vi "Settings - NI 9219.vi"(8 "Error In":errorcluster) -> (0 "Error Out":errorcluster={"status"=TRUE, "code"=-200077, "source"="Property Node DAQmx Channel (arg 2) in DAQmx Create Channel (AI-Temperature-Thermocouple).vi:1->Settings - NI 9211.vi <append>\n<B>Property: </B>AI.Temp.Units\n<B>Requested Value: </B>\n<B>You Can Select: </B>Deg C, Deg F, Kelvins, Deg R, From Custom Scale\n\n<B>Channel Name: </B>Temperature\n\n<B>Task Name: </B>_unnamedTask<E>"}, 3 "Cancelled?":bool)   [LabVIEW 2011]
doc: "This VI will get settings for NI 9211 measurement."
uses:
  SubVIs/Controls/4ch.ctl
  SubVIs/Controls/TransparencyEffectOperations.ctl
  <vilib>/DAQmx/create/channels.llb/DAQmx Create Channel (AI-Temperature-Thermocouple).vi
  <vilib>/DAQmx/configure/timing.llb/DAQmx Timing (Sample Clock).vi
  Program Files/National Instruments/LabVIEW 2011/resource/objmgr/daqmx.rc
panel:
  in  "NR of Samples":i32=3
  in  "Sample Mode":i32(ring)=10123 items=["Finite Samples"=10178, "Continuous Samples"=10123, "Hardware Timed Single Point"=12522]
  in  "Rate":dbl=10.0
  in  "Unit":i32(ring)=10143 items=["Deg C"=10143, "Deg F"=10144, "Kelvins"=10325, "Deg R"=10145, "From Custom Scale"=10065]
  in  "Thermocouple Type":i32(ring)=10072 items=["J"=10072, "K"=10073, "N"=10077, "R"=10082, "S"=10085, "T"=10086, "B"=10047, "E"=10055]
  in  "CJC source":i32(ring)=10200 items=["Built-In"=10200, "Constant Value"=10116, "Channel"=10113]
  in  "Channel":T1
  in  "Min":dbl=10.0
  in  "Max":dbl=40.0
  in  "Header For Measurement File":string="Temperature CH0"
  in  "Cancel Button":bool
  in  "OK Button":bool
  # "NI 9219"
  # "Meas File Settings"
  # "Hardware Settings"
  # "Signal Input Range"
  # "Scaled Units"
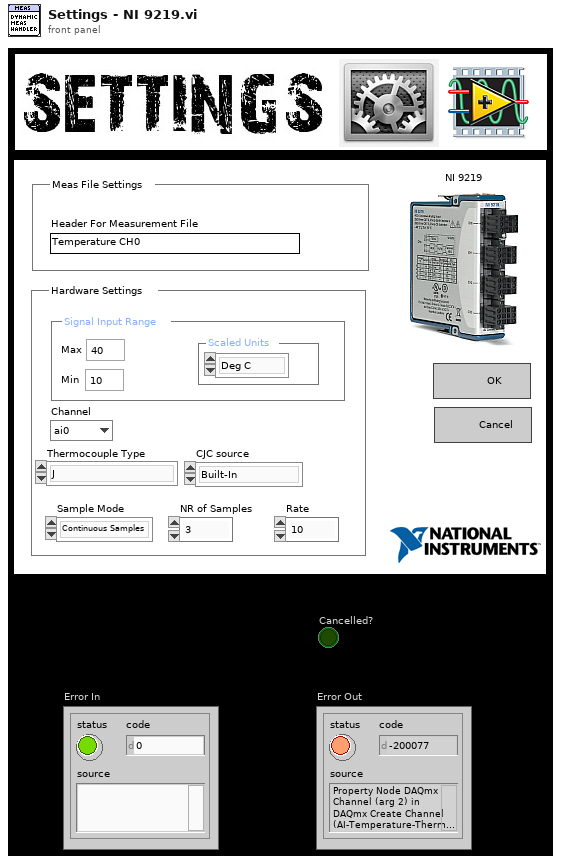
[diagram p1: front panel]
types:
  T1 = typedef "4ch.ctl" = enum16{"ai0", "ai1", "ai2", "ai3"}
  T2 = typedef "TransparencyEffectOperations.ctl" = enum16{"Show", "Hide 80%", "Hide All"}
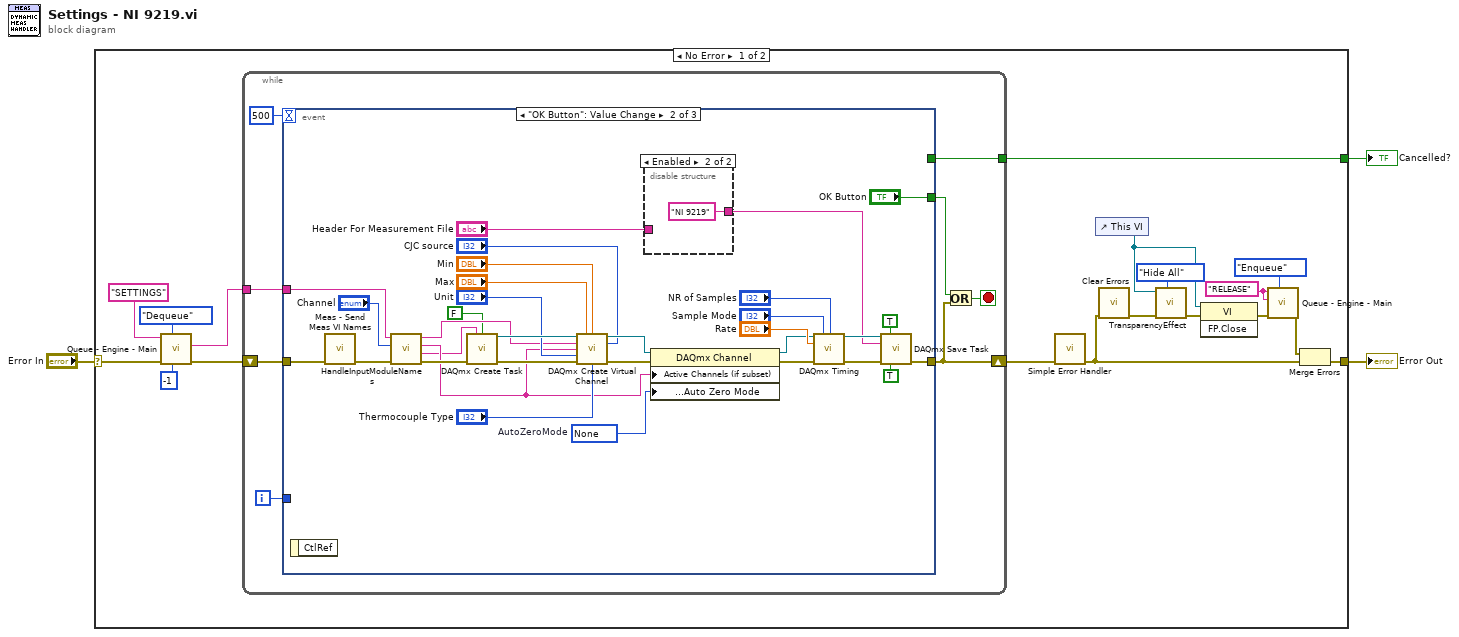
[diagram p0: block diagram]
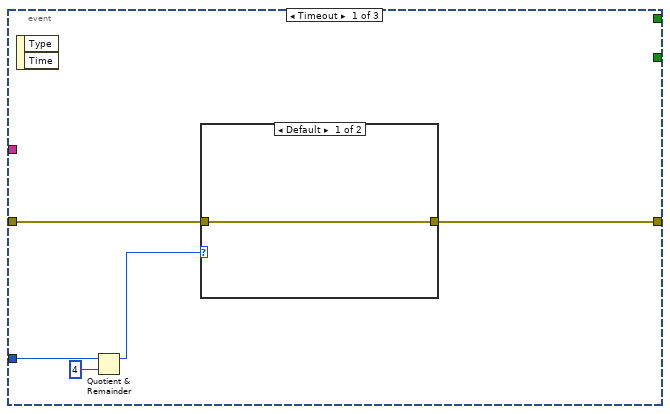
[diagram p2: hidden frame]
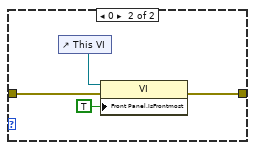
[diagram p3: hidden frame]
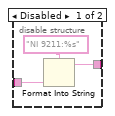
[diagram p4: hidden frame]
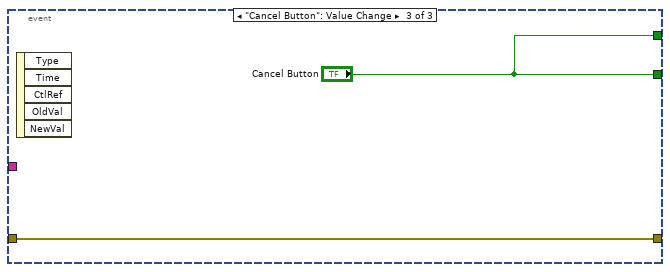
[diagram p5: hidden frame]
diagram:
  n1 = case shown="No Error" "Error In" {
    selector: "Error In" -> [w18 w78]
    tunnel: [w21 _] -> w3
    tunnel: [w4 w78] -> w2
    frame No Error {
      w10 = "RELEASE" ("Queue Data In")
      n2 = call "Queue - Engine - Main.vi"("timeout in ms (-1)"=-1, "Operation"=enum16{"Enqueue", "Dequeue", "Flush", "Release"}."Dequeue", "error in"=w18, "Queue Name In"="SETTINGS") -> ("error out"=w17:errorcluster, "Data Out"=w16:string)  [unwired: 5 in, 1 out]
      n3 = while {
        tunnel: [w29] -> w21
        shift-right: [w24] -> w5
        shift-left: w17 -> [w28]
        tunnel: w16 -> [w27]
        i -> [w25]
        stop <- w22 stop-if-true
        n4 = event shown="[1] \"OK Button\": Value Change" {
          selector: _ -> [_ _ _]
          dyn-events: _ -> [_ _ _]
          timeout: 500 -> [_ _ _]
          tunnel: [_ "OK Button" "Cancel Button"] -> w23
          tunnel: [_ _ "Cancel Button"] -> w29
          tunnel: [w33 w43 w76] -> w24
          tunnel: w28 -> [w34 w48 w76]
          tunnel: w27 -> [_ w60 _]
          tunnel: w25 -> [w32 _ _]
          event Timeout {
            n5 = event-data() -> ()  [unwired: 1 in, 2 out]
            n6 = Quotient & Remainder(x=w32, y=4) -> (x-y*floor(x/y)=w30:i32)  [unwired: 1 out]
            n7 = case shown="Default" w30 {
              tunnel: w34 -> [w35 w38]
              tunnel: [w35 w37] -> w33
              frame Default {
              }
              frame 0 {
                n8 = control-ref of="This VI"() -> (w39:refnum<vi>)
                n9 = property class="VI"(reference=w39, error in=w38, "Front Panel.IsFrontmost"=TRUE ("Front Panel Window:Is Frontmost")) -> (error out=w37:errorcluster)  [unwired: 1 out]
              }
            }
          }
          event "OK Button": Value Change {
            w69 = 10230 items=["None"=10230, "Once"=10244, "Every Sample"=10164]  # AutoZeroMode
            n10 = event-data() -> ()  [unwired: 1 in, 1 out]
            n11 = call "Meas - Send Meas VI Names.vi"("Error In"=w48) -> ("Error Out"=w47:errorcluster)  [unwired: 10 in]
            n12 = call "HandleInputModuleNames.vi"("Error In"=w47, "Channel"="Channel", "Data In"=w60) -> ("Error Out"=w62:errorcluster, "Meas Name"=w57:string, "Module and CH"=w59:string, "Channel"=w61:string)  [unwired: 5 in]
            n13 = call <vilib>:"DAQmx Create Task.vi"("new task name"=w57, "auto cleanup"=FALSE, "error in"=w62) -> ("task out"=w66:refnum<k21>, "error out"=w67:errorcluster)  [unwired: 2 in, 9 out]
            n14 = call-poly <vilib>:"DAQmx Create Virtual Channel.vi"("task in"=w66, "maximum value"="Max", "minimum value"="Min", "physical channels"=w61, "cjc source"="CJC source", "name to assign"=w59, "units"="Unit", "error in"=w67, "thermocouple type"="Thermocouple Type") -> ("task out"=w70:refnum<k21>, "error out"=w68:errorcluster)  [unwired: 4 in, 1 out]
            n15 = disable-structure shown="Enabled" {
              disable-tunnel: "Header For Measurement File" -> [w73 _]
              disable-tunnel: [w72 "NI 9219" ("Variable In")] -> w44
              frame Disabled {
                n16 = Format Into String(format string="NI 9211:%s", w73) -> (resulting string=w72:string)  [unwired: 2 in, 1 out]
              }
              frame Enabled {
              }
            }
            n17 = property class="DAQmx Channel"(reference=w70, error in=w68, "Active Channels (if subset)"=w59, "Analog Input:General Properties:Advanced:High Accuracy Settings:Auto Zero Mode"=w69) -> (reference out=w50:refnum<k21>, error out=w51:errorcluster)
            n18 = call-poly <vilib>:"DAQmx Timing.vi"("task/channels in"=w50, "sample mode"="Sample Mode", "samples per channel"="NR of Samples", "rate"="Rate", "error in"=w51) -> ("task out"=w45:refnum<k21>, "error out"=w42:errorcluster)  [unwired: 2 in, 7 out]
            n19 = call <vilib>:"DAQmx Save Task.vi"("task/channels in"=w45, "allow interactive editing?"=TRUE, "save as"=w44, "error in"=w42, "overwrite existing task?"=TRUE) -> ("error out"=w43:errorcluster)  [unwired: 9 in, 1 out]
          }
          event "Cancel Button": Value Change {
            n20 = event-data() -> ()  [unwired: 1 in, 5 out]
          }
        }
        n21 = Or(x=w23, y=w24) -> (x .or. y?=w22:bool)
      }
      n22 = call <vilib>:"Simple Error Handler.vi"("error in (no error)"=w5) -> ("error out"=w7:errorcluster)  [unwired: 4 in, 4 out]
      n23 = control-ref of="This VI"() -> (w14:refnum<vi>)
      n24 = call <vilib>:"Clear Errors.vi"("error in (no error)"=w7) -> ("error out"=w6:errorcluster)  [unwired: 6 in]
      n25 = call "TransparencyEffect.vi"("Operation"=TransparencyEffectOperations."Hide All", "error in"=w6, "VI Ref in"=w14) -> ("error out"=w11:errorcluster)  [unwired: 8 in]
      n26 = invoke class="VI" method="FP.Close"(reference=w14, error in=w11) -> (error out=w8:errorcluster)  [unwired: 1 in, 2 out]
      n27 = call "Queue - Engine - Main.vi"("Operation"=enum16{"Enqueue", "Dequeue", "Flush", "Release"}."Enqueue", "error in"=w8, "Queue Data In"=w10, "Queue Name In"=w10) -> ("error out"=w9:errorcluster)  [unwired: 5 in, 2 out]
      n28 = Merge Errors(w9, w7) -> (w4:errorcluster)
    }
    frame Error {
    }
  }
  "Cancelled?" <- w3
  "Error Out" <- w2
